vi "Register Event Callbacks.vi"(8 "error in (no error)":errorcluster, 11 "TwinCAT ADS in":refnum<class "TwinCAT ADS.lvclass">) -> (0 "error out":errorcluster, 3 "TwinCAT ADS out":refnum<class "TwinCAT ADS.lvclass">)   [LabVIEW 2018, in "TwinCAT ADS.lvclass"]
uses:
  TwinCAT ADS.lvclass
  TwinCAT ADS.lvclass/TwinCAT ADS.ctl
  TwinCAT.Ads
  Controls/ADS Notification Callback User Parameter.ctl
  Controls/Notifcation User Event.ctl
  Controls/ADS Notification Event Data.ctl
  Controls/Symbol Information.ctl
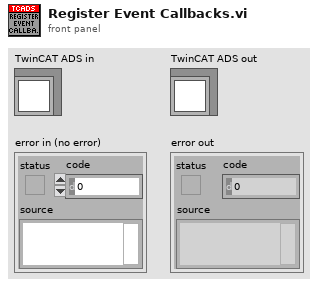
[diagram p1: front panel]
types:
  T1 = typedef "TwinCAT ADS.lvclass/ADS Notification Callback User Parameter.ctl" = cluster{"TwinCAT ADS":refnum<class "TwinCAT ADS.lvclass">, "Notification User Event ":T2}
  T2 = typedef "TwinCAT ADS.lvclass/Notifcation User Event.ctl" = refnum<user-event>
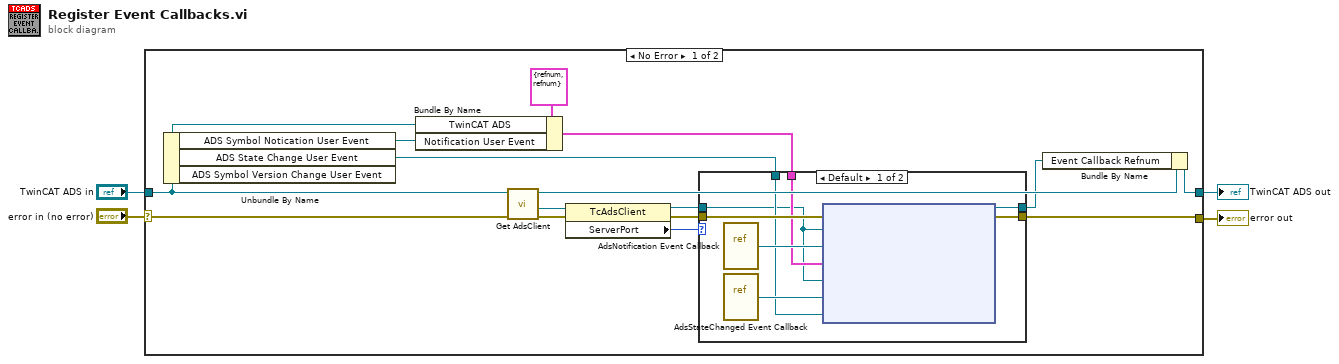
[diagram p0: block diagram]
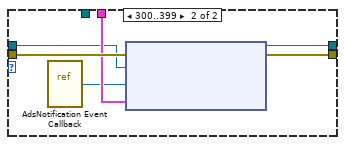
[diagram p2: hidden frame]
diagram:
  n1 = case shown="No Error" "error in (no error)" {
    selector: "error in (no error)" -> [w10 w34]
    tunnel: "TwinCAT ADS in" -> [w14 w35]
    tunnel: [w17 w35] -> w3
    tunnel: [w16 w34] -> w2
    frame No Error {
      n2 = Unbundle By Name(w14) -> ("ADS Symbol Notication User Event"=w15:refnum<user-event>, "ADS State Change User Event"=w11:refnum<user-event>)  [unwired: 1 out]
      n3 = Bundle By Name(cluster=T1 {"TwinCAT ADS"=refnum, "Notification User Event "=refnum} ("User Parameter"), "TwinCAT ADS"=w14, "Notification User Event"=w15) -> (w12:T1)
      n4 = call "Get AdsClient.vi"("error in (no error)"=w10, "TwinCAT ADS in"=w14) -> ("error out"=w9:errorcluster, ".NET TcAdsClient"=w8:refnum<k24>, "TwinCAT ADS out"=w18:refnum<class "TwinCAT ADS.lvclass">)  [unwired: 7 in]
      n5 = property class="TcAdsClient"(reference=w8, error in=w9) -> (reference out=w7:refnum<k24>, error out=w5:errorcluster, "ServerPort"=w6:i32)
      n6 = case shown="Default" w6 {
        tunnel: [w26 w33] -> w16
        tunnel: [w24 w32] -> w13
        tunnel: w12 -> [w22 w30]
        tunnel: w11 -> [w21 _]
        tunnel: w7 -> [w20 w28]
        tunnel: w5 -> [w27 w31]
        frame Default {
          n7 = vi-ref "AdsNotification Event Callback.vi"() -> ("vi reference"=w23:refnum<vi>)
          n8 = vi-ref "AdsStateChanged Event Callback.vi"() -> ("vi reference"=w25:refnum<vi>)
          n9 = node(w27, w20, w23, w22, w20, w25, w21) -> (w24:refnum<k27>, w26:errorcluster)  [unwired: 1 in]
        }
        frame 300..399 {
          n10 = vi-ref "AdsNotification Event Callback.vi"() -> ("vi reference"=w29:refnum<vi>)
          n11 = node(w31, w28, w29, w30) -> (w32:refnum<k27>, w33:errorcluster)  [unwired: 1 in]
        }
      }
      n12 = Bundle By Name(cluster=w18, "Event Callback Refnum"=w13) -> (w17:refnum<class "TwinCAT ADS.lvclass">)
    }
    frame Error {
    }
  }
  "error out" <- w2
  "TwinCAT ADS out" <- w3
